vi "CTRE_PigeonIMU_Open_TalonSRX.vi"(8 "error in":errorcluster, 10 "CAN Talon SRX Ref":T1={"DeviceStatus"={"status"=FALSE, "code"=0, "source"=""}, "Type"=enum."PWM", "PWM"={"PWM Channel"=enum."PWM 1", "DeadBand"={"Name"="", "maxPositivePwm"=0, "minPositivePwm"=0, "centerPwm"=0, "maxNegativePwm"=0, "minNegativePwm"=0, "angularRange"=0}}, "CAN"={"Device Number"=0, "SetOutput VI Ref"=variant(enum8{"Percent VBus", "Current", "Speed", "Position", "Voltage"} enum."Percent VBus"), "GetOutput VI Ref"=variant(refnum<k1> refnum), "Enable VI Ref"=variant(dbl 12.0), "Disable VI Ref"=variant(enum8{"Percent VBus", "Speed", "Position", "Slave", "Unchanged / Invalid", "Voltage Compensation", "Current", "Motion Profile"} enum."Percent VBus"), "Data"=variant}, "Invert"=FALSE}) -> (0 "error out":errorcluster, 3 "PigeonIMUDevRef":T5={"DeviceStatus"={"status"=FALSE, "code"=0, "source"=""}, "Device Number"=0, "Type"=352321536, "Device ID"=0} {"Type" items=["CAN"=352321536, "TalonSRX"=33554432]})   [LabVIEW 2016]
doc: "Opens a Pigeon IMU Device Reference using the Device Reference from a Talon SRX."
uses:
  <vilib>/Rock Robotics/WPI/ThirdParty/Sensors/Pigeon IMU/CTRE_PigeonIMU_DeviceRef.ctl
  <vilib>/Rock Robotics/WPI/ThirdParty/Sensors/Pigeon IMU/CTRE_PigeonIMU_ConnectionType.ctl
  <vilib>/Rock Robotics/WPI/MotorControl/WPI_MotorControlDeviceRef.ctl
  <vilib>/Rock Robotics/WPI/MotorControl/WPI_MotorControlType.ctl
  <vilib>/Rock Robotics/SystemInterfaces/DIO/FPGA_DIOPWMChannel.ctl
  <vilib>/Rock Robotics/WPI/PWM/WPI_PWMDeadband.ctl
  <vilib>/Rock Robotics/WPI/ThirdParty/Sensors/Pigeon IMU/CTRE_PigeonIMU_MessageIDs.ctl
  <vilib>/Rock Robotics/WPI/ThirdParty/Sensors/Pigeon IMU/CTRE_PigeonIMU_UsageTypes.ctl
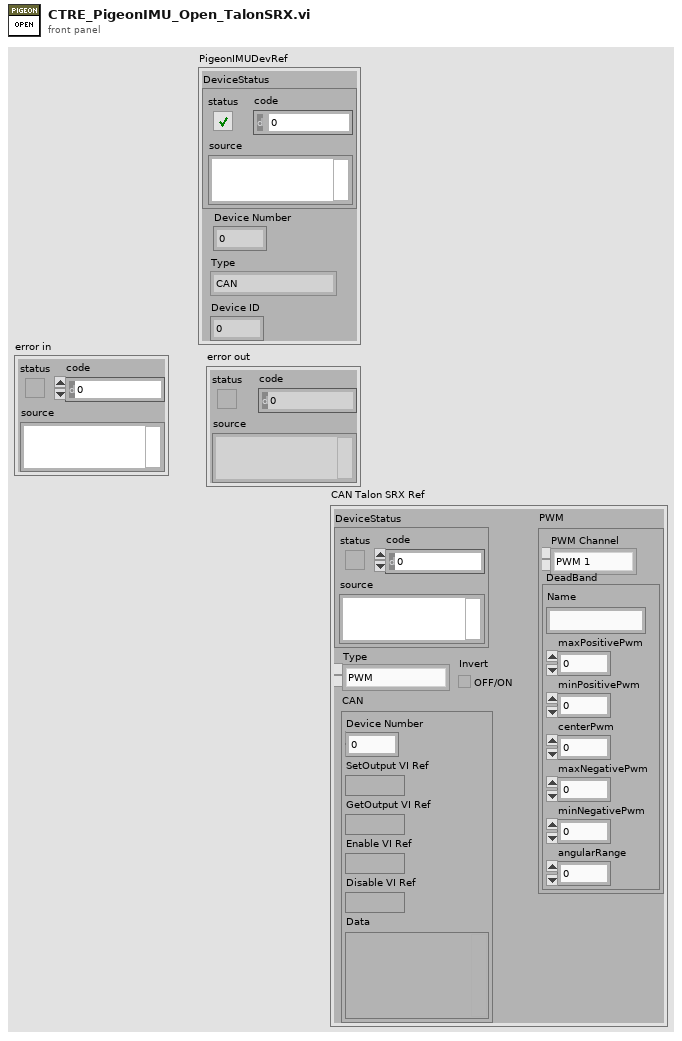
[diagram p1: front panel]
types:
  T1 = typedef "WPI_MotorControlDeviceRef.ctl" = cluster{"DeviceStatus":errorcluster, "Type":T2, "PWM":cluster{"PWM Channel":T3, "DeadBand":T4}, "CAN":cluster{"Device Number":u8, "SetOutput VI Ref":variant, "GetOutput VI Ref":variant, "Enable VI Ref":variant, "Disable VI Ref":variant, "Data":variant}, "Invert":bool}
  T2 = typedef "WPI_MotorControlType.ctl" = enum16{"PWM", "CAN"}
  T3 = typedef "FPGA_DIOPWMChannel.ctl" = enum8{"PWM 0", "PWM 1", "PWM 2", "PWM 3", "PWM 4", "PWM 5", "PWM 6", "PWM 7", "PWM 8", "PWM 9", "PWM MXP 0", "PWM MXP 1", "PWM MXP 2", "PWM MXP 3", "PWM MXP 4", "PWM MXP 5", "PWM MXP 6", "PWM MXP 7", "PWM MXP 8", "PWM MXP 9", "Invalid"}
  T4 = typedef "WPI_PWMDeadband.ctl" = cluster{"Name":string, "maxPositivePwm":i32, "minPositivePwm":i32, "centerPwm":i32, "maxNegativePwm":i32, "minNegativePwm":i32, "angularRange":u16}
  T5 = typedef "CTRE_PigeonIMU_DeviceRef.ctl" = cluster{"DeviceStatus":errorcluster, "Device Number":u8, "Type":T6, "Device ID":u32}
  T6 = typedef "CTRE_PigeonIMU_ConnectionType.ctl" = u32
  T7 = typedef "CTRE_PigeonIMU_UsageTypes.ctl" = u32
  T8 = typedef "CTRE_PigeonIMU_MessageIDs.ctl" = u32
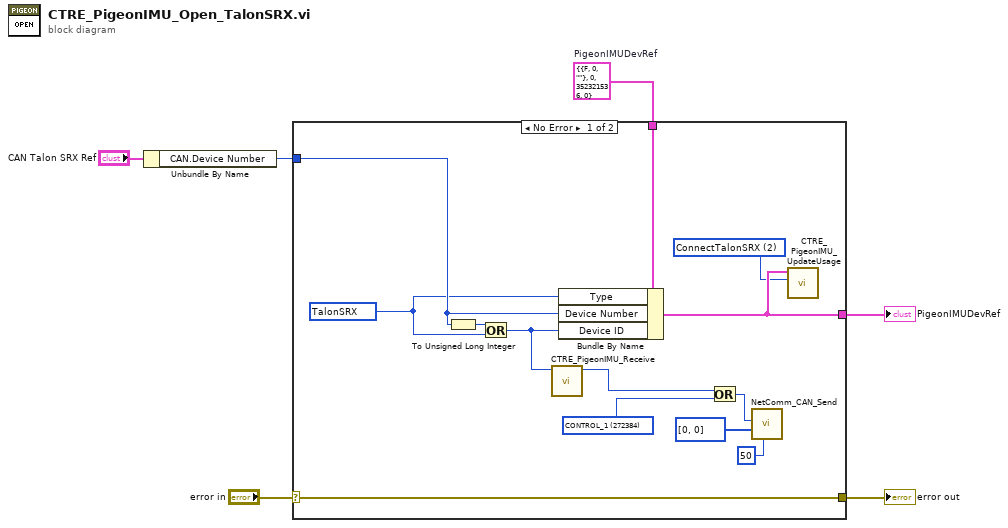
[diagram p0: block diagram]
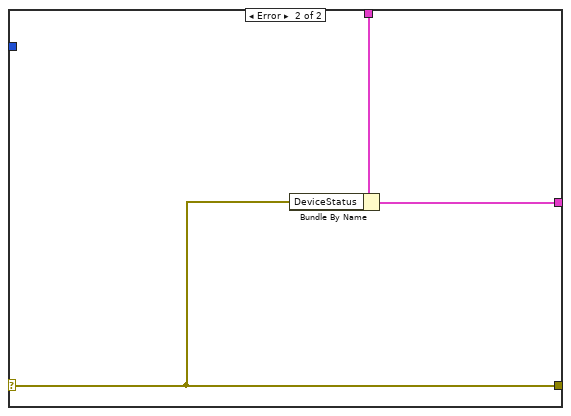
[diagram p2: hidden frame]
diagram:
  w4 = T5 {"DeviceStatus"={"status"=FALSE, "code"=0, "source"=""}, "Device Number"=0, "Type"=352321536, "Device ID"=0}  # PigeonIMUDevRef
  n1 = Unbundle By Name("CAN Talon SRX Ref") -> ("CAN.Device Number"=w1:u8)
  n2 = case shown="No Error" "error in" {
    selector: "error in" -> [w19 w21]
    tunnel: [w19 w21] -> w5
    tunnel: w4 -> [w18 w22]
    tunnel: [w8 w20] -> w3
    tunnel: w1 -> [w16 _]
    frame No Error {
      w7 = T7 2 items=["Defaul"=0, "ConnectCAN"=1, "ConnectTalonSRX"=2, "GetCompass"=134217728, "GetYPR"=268435456, "GetFused"=536870912, "GetAccel"=1073741824, "TempComp"=2147483648] ("Usage")
      w9 = T6 33554432 items=["CAN"=352321536, "TalonSRX"=33554432] ("Connection Type")
      w15 = T8 272384 items=["RAW_STATUS_2"=265280, "RAW_STATUS_4"=265408, "RAW_STATUS_6"=265536, "BIASED_STATUS_2"=269376, "BIASED_STATUS_4"=269504, "BIASED_STATUS_6"=269632, "COND_STATUS_1"=270336, "COND_STATUS_2"=270400, "COND_STATUS_3"=270464, "COND_STATUS_4"=270528, "COND_STATUS_5"=270592, "COND_STATUS_6"=270656, "COND_STATUS_7"=270720, "COND_STATUS_8"=270784, "COND_STATUS_9"=270848, "COND_STATUS_10"=270912, "CONTROL_1"=272384, "PARAM_REQUEST"=273408, "PARAM_RESPONSE"=273472, "PARAM_SET"=273536] ("MessageIDs")
      n3 = To Unsigned Long Integer(number=w16) -> (unsigned 32bit integer=w17:u32)
      n4 = Or(x=w17, y=w9) -> (x .or. y?=w11:T6)
      n5 = call <vilib>:"CTRE_PigeonIMU_Receive.vi"("Device ID"=w11) -> ("Device ID Out"=w10:u32)  [unwired: 10 in]
      n6 = Bundle By Name(cluster=w18, "Type"=w9, "Device Number"=w16, "Device ID"=w11) -> (w8:T5)
      n7 = Or(x=w10, y=w15) -> (x .or. y?=w14:T8)
      n8 = call <vilib>:"NetComm_CAN_Send.vi"("Period (ms)"=50, "Data"=u8[] [0, 0], "Message ID"=w14) -> ()  [unwired: 8 in, 1 out]
      n9 = call <vilib>:"CTRE_PigeonIMU_UpdateUsage.vi"("Usage"=w7, "PigeonIMUDevRef"=w8) -> ()  [unwired: 10 in]
    }
    frame Error {
      n10 = Bundle By Name(cluster=w22, "DeviceStatus"=w21) -> (w20:T5)
    }
  }
  "error out" <- w5
  "PigeonIMUDevRef" <- w3
